vi "SUB-FILE-Measurement data_Save.vi"(0 "File Server Path":string="C:\\InLCT\\Measurement Data\\WB1", 1 "File Name":string="C:\\InLCT\\Measurement Data\\WB1", 2 "배열-열헤더":string[](array[string])=["1", "1", "1", "1", "1", "1", "1", "1"], 3 "배열-Data":dbl[][](array[numeric])=[[30.4, 28.4, 28.4, 28.4, 28.4, 28.4, 28.4, 28.4, 28.4, 28.4, 28.4, 28.4, 28.4, 28.4, 28.4, 28.4, 28.4, 28.4, 28.4, 28.4, 28.4, 28.4, 28.4, 28.4, 28.4, 28.4, 28.4, 28.4, 28.4, 28.4, 28.4, 28.4, 28.4, 28.4, 28.4, 28.4, 28.4, 28.4, 28.4, 28.4, 28.4, 28.4, 28.4, 28.4, 28.4, 28.4, 28.4, 28.4, 28.4, 28.4, 28.4, 28.4, 28.4, 28.4, 28.4, 28.4, 28.4, 28.4, 28.4, 28.4, 28.4, 28.4, 28.4, 28.4, 28.4, 28.4, 28.4, 28.4, 28.4, 28.4, 28.4, 28.4, 28.4, 28.4, 28.4, 28.4, 28.4, 28.4, 28.4, 28.4, 28.4, 28.4, 28.4, 28.4, 28.4, 28.4, 28.4, 28.4, 28.4, 28.4, 28.4, 28.4, 28.4, 28.4, 28.4, 28.4, 28.4, 28.4, 28.4, 28.4, 28.4, 28.4, 28.4, 28.4, 28.4, 28.4, 28.4, 28.4, 28.4, 28.4, 28.4, 28.4, 28.4, 28.4, 28.4, 28.4, 28.4, 28.4, 28.4, 28.4, 28.4, 28.4, 28.4, 28.4, 28.4, 28.4, 28.4, 28.4, 28.4, 28.4, 28.4, 28.4, 28.4, 28.4, 28.4, 28.4, 28.4, 28.4, 28.4, 28.4, 28.4, 28.4, 28.4, 28.4, 28.4, 28.4, 28.4, 28.4, 28.4, 28.4, 28.4, 28.4, 28.4, 28.4, 28.4, 28.4, 28.4, 28.4, 28.4, 28.4, 28.4, 28.4, 28.4, 28.4, 28.4, 28.4, 28.4, 28.4, 28.4, 28.4, 28.4, 28.4, 28.4, 28.4, 28.4, 28.4, 28.4, 28.4, 28.4, 28.4, 28.4, 28.4, 28.4, 28.4, 28.4, 28.4, 28.4, 28.4, 28.4, 28.4, 28.4, 28.4, 28.4, 28.4, 28.4, 28.4, 28.4, 28.4, 28.4, 28.4, 28.4, 28.4, 28.4, 28.4, 28.4, 28.4, 28.4, 28.4, 28.4, 28.4, 28.4, 28.4, 28.4, 28.4, 28.4, 28.4, 28.4, 28.4, 28.4, 28.4, 28.4, 28.4, 28.4, 28.4, 28.4, 28.4, 28.4, 28.4, 28.4, 28.4, 28.4, 28.4, 28.4, 28.4, 28.4, 28.4, 28.4, 28.4, 28.4, 28.4, 28.4, 28.4, 28.4, 28.4, 28.4, 28.4, 28.4, 28.4, 28.4, 28.4, 28.4, 28.4, 28.4, 28.4, 28.4, 28.4, 28.4, 28.4, 28.4, 28.4, 28.4, 28.4, 28.4, 28.4, 28.4, 28.4, 28.4, 28.4, 28.4, 28.4, 28.4, 28.4, 28.4, 28.4, 28.4, 28.4, 28.4, 28.4, 28.4, 28.4, 28.4, 28.4, 28.4, 28.4, 28.4, 28.4, 28.4, 28.4], [28.4, 28.4, 28.4, 28.4, 28.4, 28.4, 28.4, 28.4, 28.4, 28.4, 28.4, 28.4, 28.4, 28.4, 28.4, 28.4, 28.4, 28.4, 28.4, 28.4, 28.4, 28.4, 28.4, 28.4, 28.4, 28.4, 28.4, 28.4, 28.4, 28.4, 28.4, 28.4, 28.4, 28.4, 28.4, 28.4, 28.4, 28.4, 28.4, 28.4, 28.4, 28.4, 28.4, 28.4, 28.4, 28.4, 28.4, 28.4, 28.4, 28.4, 28.4, 28.4, 28.4, 28.4, 28.4, 28.4, 28.4, 28.4, 28.4, 28.4, 28.4, 28.4, 28.4, 28.4, 28.4, 28.4, 28.4, 28.4, 28.4, 28.4, 28.4, 28.4, 28.4, 28.4, 28.4, 28.4, 28.4, 28.4, 28.4, 28.4, 28.4, 28.4, 28.4, 28.4, 28.4, 28.4, 28.4, 28.4, 28.4, 28.4, 28.4, 28.4, 28.4, 28.4, 28.4, 28.4, 28.4, 28.4, 28.4, 28.4, 28.4, 28.4, 28.4, 28.4, 28.4, 28.4, 28.4, 28.4, 28.4, 28.4, 28.4, 28.4, 28.4, 28.4, 28.4, 28.4, 28.4, 28.4, 28.4, 28.4, 28.4, 28.4, 28.4, 28.4, 28.4, 28.4, 28.4, 28.4, 28.4, 28.4, 28.4, 28.4, 28.4, 28.4, 28.4, 28.4, 28.4, 28.4, 28.4, 28.4, 28.4, 28.4, 28.4, 28.4, 28.4, 28.4, 28.4, 28.4, 28.4, 28.4, 28.4, 28.4, 28.4, 28.4, 28.4, 28.4, 28.4, 28.4, 28.4, 28.4, 28.4, 28.4, 28.4, 28.4, 28.4, 28.4, 28.4, 28.4, 28.4, 28.4, 28.4, 28.4, 28.4, 28.4, 28.4, 28.4, 28.4, 28.4, 28.4, 28.4, 28.4, 28.4, 28.4, 28.4, 28.4, 28.4, 28.4, 28.4, 28.4, 28.4, 28.4, 28.4, 28.4, 28.4, 28.4, 28.4, 28.4, 28.4, 28.4, 28.4, 28.4, 28.4, 28.4, 28.4, 28.4, 28.4, 28.4, 28.4, 28.4, 28.4, 28.4, 28.4, 28.4, 28.4, 28.4, 28.4, 28.4, 28.4, 28.4, 28.4, 28.4, 28.4, 28.4, 28.4, 28.4, 28.4, 28.4, 28.4, 28.4, 28.4, 28.4, 28.4, 28.4, 28.4, 28.4, 28.4, 28.4, 28.4, 28.4, 28.4, 28.4, 28.4, 28.4, 28.4, 28.4, 28.4, 28.4, 28.4, 28.4, 28.4, 28.4, 28.4, 28.4, 28.4, 28.4, 28.4, 28.4, 28.4, 28.4, 28.4, 28.4, 28.4, 28.4, 28.4, 28.4, 28.4, 28.4, 28.4, 28.4, 28.4, 28.4, 28.4, 28.4, 28.4, 28.4, 28.4, 28.4, 28.4, 28.4, 28.4, 28.4, 28.4, 28.4, 28.4, 28.4, 28.4, 28.4, 28.4], [28.4, 28.4, 28.4, 28.4, 28.4, 28.4, 28.4, 28.4, 28.4, 28.4, 28.4, 28.4, 28.4, 28.4, 28.4, 28.4, 28.4, 28.4, 28.4, 28.4, 28.4, 28.4, 28.4, 28.4, 28.4, 28.4, 28.4, 28.4, 28.4, 28.4, 28.4, 28.4, 28.4, 28.4, 28.4, 28.4, 28.4, 28.4, 28.4, 28.4, 28.4, 28.4, 28.4, 28.4, 28.4, 28.4, 28.4, 28.4, 28.4, 28.4, 28.4, 28.4, 28.4, 28.4, 28.4, 28.4, 28.4, 28.4, 28.4, 28.4, 28.4, 28.4, 28.4, 28.4, 28.4, 28.4, 28.4, 28.4, 28.4, 28.4, 28.4, 28.4, 28.4, 28.4, 28.4, 28.4, 28.4, 28.4, 28.4, 28.4, 28.4, 28.4, 28.4, 28.4, 28.4, 28.4, 28.4, 28.4, 28.4, 28.4, 28.4, 28.4, 28.4, 28.4, 28.4, 28.4, 28.4, 28.4, 28.4, 28.4, 28.4, 28.4, 28.4, 28.4, 28.4, 28.4, 28.4, 28.4, 28.4, 28.4, 28.4, 28.4, 28.4, 28.4, 28.4, 28.4, 28.4, 28.4, 28.4, 28.4, 28.4, 28.4, 28.4, 28.4, 28.4, 28.4, 28.4, 28.4, 28.4, 28.4, 28.4, 28.4, 28.4, 28.4, 28.4, 28.4, 28.4, 28.4, 28.4, 28.4, 28.4, 28.4, 28.4, 28.4, 28.4, 28.4, 28.4, 28.4, 28.4, 28.4, 28.4, 28.4, 28.4, 28.4, 28.4, 28.4, 28.4, 28.4, 28.4, 28.4, 28.4, 28.4, 28.4, 28.4, 28.4, 28.4, 28.4, 28.4, 28.4, 28.4, 28.4, 28.4, 28.4, 28.4, 28.4, 28.4, 28.4, 28.4, 28.4, 28.4, 28.4, 28.4, 28.4, 28.4, 28.4, 28.4, 28.4, 28.4, 28.4, 28.4, 28.4, 28.4, 28.4, 28.4, 28.4, 28.4, 28.4, 28.4, 28.4, 28.4, 28.4, 28.4, 28.4, 28.4, 28.4, 28.4, 28.4, 28.4, 28.4, 28.4, 28.4, 28.4, 28.4, 28.4, 28.4, 28.4, 28.4, 28.4, 28.4, 28.4, 28.4, 28.4, 28.4, 28.4, 28.4, 28.4, 28.4, 28.4, 28.4, 28.4, 28.4, 28.4, 28.4, 28.4, 28.4, 28.4, 28.4, 28.4, 28.4, 28.4, 28.4, 28.4, 28.4, 28.4, 28.4, 28.4, 28.4, 28.4, 28.4, 28.4, 28.4, 28.4, 28.4, 28.4, 28.4, 28.4, 28.4, 28.4, 28.4, 28.4, 28.4, 28.4, 28.4, 28.4, 28.4, 28.4, 28.4, 28.4, 28.4, 28.4, 28.4, 28.4, 28.4, 28.4, 28.4, 28.4, 28.4, 28.4, 28.4, 28.4, 28.4, 28.4, 28.4, 28.4, 28.4, 28.4, 28.4, 28.4], [28.4, 28.4, 28.4, 28.4, 28.4, 28.4, 28.4, 28.4, 28.4, 28.4, 28.4, 28.4, 28.4, 28.4, 28.4, 28.4, 28.4, 28.4, 28.4, 28.4, 28.4, 28.4, 28.4, 28.4, 28.4, 28.4, 28.4, 28.4, 28.4, 28.4, 28.4, 28.4, 28.4, 28.4, 28.4, 28.4, 28.4, 28.4, 28.4, 28.4, 28.4, 28.4, 28.4, 28.4, 28.4, 28.4, 28.4, 28.4, 28.4, 28.4, 28.4, 28.4, 28.4, 28.4, 28.4, 28.4, 28.4, 28.4, 28.4, 28.4, 28.4, 28.4, 28.4, 28.4, 28.4, 28.4, 28.4, 28.4, 28.4, 28.4, 28.4, 28.4, 28.4, 28.4, 28.4, 28.4, 28.4, 28.4, 28.4, 28.4, 28.4, 28.4, 28.4, 28.4, 28.4, 28.4, 28.4, 28.4, 28.4, 28.4, 28.4, 28.4, 28.4, 28.4, 28.4, 28.4, 28.4, 28.4, 28.4, 28.4, 28.4, 28.4, 28.4, 28.4, 28.4, 28.4, 28.4, 28.4, 28.4, 28.4, 28.4, 28.4, 28.4, 28.4, 28.4, 28.4, 28.4, 28.4, 28.4, 28.4, 28.4, 28.4, 28.4, 28.4, 28.4, 28.4, 28.4, 28.4, 28.4, 28.4, 28.4, 28.4, 28.4, 28.4, 28.4, 28.4, 28.4, 28.4, 28.4, 28.4, 28.4, 28.4, 28.4, 28.4, 28.4, 28.4, 28.4, 28.4, 28.4, 28.4, 28.4, 28.4, 28.4, 28.4, 28.4, 28.4, 28.4, 28.4, 28.4, 28.4, 28.4, 28.4, 28.4, 28.4, 28.4, 28.4, 28.4, 28.4, 28.4, 28.4, 28.4, 28.4, 28.4, 28.4, 28.4, 28.4, 28.4, 28.4, 28.4, 28.4, 28.4, 28.4, 28.4, 28.4, 28.4, 28.4, 28.4, 28.4, 28.4, 28.4, 28.4, 28.4, 28.4, 28.4, 28.4, 28.4, 28.4, 28.4, 28.4, 28.4, 28.4, 28.4, 28.4, 28.4, 28.4, 28.4, 28.4, 28.4, 28.4, 28.4, 28.4, 28.4, 28.4, 28.4, 28.4, 28.4, 28.4, 28.4, 28.4, 28.4, 28.4, 28.4, 28.4, 28.4, 28.4, 28.4, 28.4, 28.4, 28.4, 28.4, 28.4, 28.4, 28.4, 28.4, 28.4, 28.4, 28.4, 28.4, 28.4, 28.4, 28.4, 28.4, 28.4, 28.4, 28.4, 28.4, 28.4, 28.4, 28.4, 28.4, 28.4, 28.4, 28.4, 28.4, 28.4, 28.4, 28.4, 28.4, 28.4, 28.4, 28.4, 28.4, 28.4, 28.4, 28.4, 28.4, 28.4, 28.4, 28.4, 28.4, 28.4, 28.4, 28.4, 28.4, 28.4, 28.4, 28.4, 28.4, 28.4, 28.4, 28.4, 28.4, 28.4, 28.4, 28.4, 28.4, 28.4, 28.4], [28.4, 28.4, 28.4, 28.4, 28.4, 28.4, 28.4, 28.4, 28.4, 28.4, 28.4, 28.4, 28.4, 28.4, 28.4, 28.4, 28.4, 28.4, 28.4, 28.4, 28.4, 28.4, 28.4, 28.4, 28.4, 28.4, 28.4, 28.4, 28.4, 28.4, 28.4, 28.4, 28.4, 28.4, 28.4, 28.4, 28.4, 28.4, 28.4, 28.4, 28.4, 28.4, 28.4, 28.4, 28.4, 28.4, 28.4, 28.4, 28.4, 28.4, 28.4, 28.4, 28.4, 28.4, 28.4, 28.4, 28.4, 28.4, 28.4, 28.4, 28.4, 28.4, 28.4, 28.4, 28.4, 28.4, 28.4, 28.4, 28.4, 28.4, 28.4, 28.4, 28.4, 28.4, 28.4, 28.4, 28.4, 28.4, 28.4, 28.4, 28.4, 28.4, 28.4, 28.4, 28.4, 28.4, 28.4, 28.4, 28.4, 28.4, 28.4, 28.4, 28.4, 28.4, 28.4, 28.4, 28.4, 28.4, 28.4, 28.4, 28.4, 28.4, 28.4, 28.4, 28.4, 28.4, 28.4, 28.4, 28.4, 28.4, 28.4, 28.4, 28.4, 28.4, 28.4, 28.4, 28.4, 28.4, 28.4, 28.4, 28.4, 28.4, 28.4, 28.4, 28.4, 28.4, 28.4, 28.4, 28.4, 28.4, 28.4, 28.4, 28.4, 28.4, 28.4, 28.4, 28.4, 28.4, 28.4, 28.4, 28.4, 28.4, 28.4, 28.4, 28.4, 28.4, 28.4, 28.4, 28.4, 28.4, 28.4, 28.4, 28.4, 28.4, 28.4, 28.4, 28.4, 28.4, 28.4, 28.4, 28.4, 28.4, 28.4, 28.4, 28.4, 28.4, 28.4, 28.4, 28.4, 28.4, 28.4, 28.4, 28.4, 28.4, 28.4, 28.4, 28.4, 28.4, 28.4, 28.4, 28.4, 28.4, 28.4, 28.4, 28.4, 28.4, 28.4, 28.4, 28.4, 28.4, 28.4, 28.4, 28.4, 28.4, 28.4, 28.4, 28.4, 28.4, 28.4, 28.4, 28.4, 28.4, 28.4, 28.4, 28.4, 28.4, 28.4, 28.4, 28.4, 28.4, 28.4, 28.4, 28.4, 28.4, 28.4, 28.4, 28.4, 28.4, 28.4, 28.4, 28.4, 28.4, 28.4, 28.4, 28.4, 28.4, 28.4, 28.4, 28.4, 28.4, 28.4, 28.4, 28.4, 28.4, 28.4, 28.4, 28.4, 28.4, 28.4, 28.4, 28.4, 28.4, 28.4, 28.4, 28.4, 28.4, 28.4, 28.4, 28.4, 28.4, 28.4, 28.4, 28.4, 28.4, 28.4, 28.4, 28.4, 28.4, 28.4, 28.4, 28.4, 28.4, 28.4, 28.4, 28.4, 28.4, 28.4, 28.4, 28.4, 28.4, 28.4, 28.4, 28.4, 28.4, 28.4, 28.4, 28.4, 28.4, 28.4, 28.4, 28.4, 28.4, 28.4, 28.4, 28.4, 28.4, 28.4, 28.4], [28.4, 28.4, 28.4, 28.4, 28.4, 28.4, 28.4, 28.4, 28.4, 28.4, 28.4, 28.4, 28.4, 28.4, 28.4, 28.4, 28.4, 28.4, 28.4, 28.4, 28.4, 28.4, 28.4, 28.4, 28.4, 28.4, 28.4, 28.4, 28.4, 28.4, 28.4, 28.4, 28.4, 28.4, 28.4, 28.4, 28.4, 28.4, 28.4, 28.4, 28.4, 28.4, 28.4, 28.4, 28.4, 28.4, 28.4, 28.4, 28.4, 28.4, 28.4, 28.4, 28.4, 28.4, 28.4, 28.4, 28.4, 28.4, 28.4, 28.4, 28.4, 28.4, 28.4, 28.4, 28.4, 28.4, 28.4, 28.4, 28.4, 28.4, 28.4, 28.4, 28.4, 28.4, 28.4, 28.4, 28.4, 28.4, 28.4, 28.4, 28.4, 28.4, 28.4, 28.4, 28.4, 28.4, 28.4, 28.4, 28.4, 28.4, 28.4, 28.4, 28.4, 28.4, 28.4, 28.4, 28.4, 28.4, 28.4, 28.4, 28.4, 28.4, 28.4, 28.4, 28.4, 28.4, 28.4, 28.4, 28.4, 28.4, 28.4, 28.4, 28.4, 28.4, 28.4, 28.4, 28.4, 28.4, 28.4, 28.4, 28.4, 28.4, 28.4, 28.4, 28.4, 28.4, 28.4, 28.4, 28.4, 28.4, 28.4, 28.4, 28.4, 28.4, 28.4, 28.4, 28.4, 28.4, 28.4, 28.4, 28.4, 28.4, 28.4, 28.4, 28.4, 28.4, 28.4, 28.4, 28.4, 28.4, 28.4, 28.4, 28.4, 28.4, 28.4, 28.4, 28.4, 28.4, 28.4, 28.4, 28.4, 28.4, 28.4, 28.4, 28.4, 28.4, 28.4, 28.4, 28.4, 28.4, 28.4, 28.4, 28.4, 28.4, 28.4, 28.4, 28.4, 28.4, 28.4, 28.4, 28.4, 28.4, 28.4, 28.4, 28.4, 28.4, 28.4, 28.4, 28.4, 28.4, 28.4, 28.4, 28.4, 28.4, 28.4, 28.4, 28.4, 28.4, 28.4, 28.4, 28.4, 28.4, 28.4, 28.4, 28.4, 28.4, 28.4, 28.4, 28.4, 28.4, 28.4, 28.4, 28.4, 28.4, 28.4, 28.4, 28.4, 28.4, 28.4, 28.4, 28.4, 28.4, 28.4, 28.4, 28.4, 28.4, 28.4, 28.4, 28.4, 28.4, 28.4, 28.4, 28.4, 28.4, 28.4, 28.4, 28.4, 28.4, 28.4, 28.4, 28.4, 28.4, 28.4, 28.4, 28.4, 28.4, 28.4, 28.4, 28.4, 28.4, 28.4, 28.4, 28.4, 28.4, 28.4, 28.4, 28.4, 28.4, 28.4, 28.4, 28.4, 28.4, 28.4, 28.4, 28.4, 28.4, 28.4, 28.4, 28.4, 28.4, 28.4, 28.4, 28.4, 28.4, 28.4, 28.4, 28.4, 28.4, 28.4, 28.4, 28.4, 28.4, 28.4, 28.4, 28.4, 28.4, 28.4, 28.4], [28.4, 28.4, 28.4, 28.4, 28.4, 28.4, 28.4, 28.4, 28.4, 28.4, 28.4, 28.4, 28.4, 28.4, 28.4, 28.4, 28.4, 28.4, 28.4, 28.4, 28.4, 28.4, 28.4, 28.4, 28.4, 28.4, 28.4, 28.4, 28.4, 28.4, 28.4, 28.4, 28.4, 28.4, 28.4, 28.4, 28.4, 28.4, 28.4, 28.4, 28.4, 28.4, 28.4, 28.4, 28.4, 28.4, 28.4, 28.4, 28.4, 28.4, 28.4, 28.4, 28.4, 28.4, 28.4, 28.4, 28.4, 28.4, 28.4, 28.4, 28.4, 28.4, 28.4, 28.4, 28.4, 28.4, 28.4, 28.4, 28.4, 28.4, 28.4, 28.4, 28.4, 28.4, 28.4, 28.4, 28.4, 28.4, 28.4, 28.4, 28.4, 28.4, 28.4, 28.4, 28.4, 28.4, 28.4, 28.4, 28.4, 28.4, 28.4, 28.4, 28.4, 28.4, 28.4, 28.4, 28.4, 28.4, 28.4, 28.4, 28.4, 28.4, 28.4, 28.4, 28.4, 28.4, 28.4, 28.4, 28.4, 28.4, 28.4, 28.4, 28.4, 28.4, 28.4, 28.4, 28.4, 28.4, 28.4, 28.4, 28.4, 28.4, 28.4, 28.4, 28.4, 28.4, 28.4, 28.4, 28.4, 28.4, 28.4, 28.4, 28.4, 28.4, 28.4, 28.4, 28.4, 28.4, 28.4, 28.4, 28.4, 28.4, 28.4, 28.4, 28.4, 28.4, 28.4, 28.4, 28.4, 28.4, 28.4, 28.4, 28.4, 28.4, 28.4, 28.4, 28.4, 28.4, 28.4, 28.4, 28.4, 28.4, 28.4, 28.4, 28.4, 28.4, 28.4, 28.4, 28.4, 28.4, 28.4, 28.4, 28.4, 28.4, 28.4, 28.4, 28.4, 28.4, 28.4, 28.4, 28.4, 28.4, 28.4, 28.4, 28.4, 28.4, 28.4, 28.4, 28.4, 28.4, 28.4, 28.4, 28.4, 28.4, 28.4, 28.4, 28.4, 28.4, 28.4, 28.4, 28.4, 28.4, 28.4, 28.4, 28.4, 28.4, 28.4, 28.4, 28.4, 28.4, 28.4, 28.4, 28.4, 28.4, 28.4, 28.4, 28.4, 28.4, 28.4, 28.4, 28.4, 28.4, 28.4, 28.4, 28.4, 28.4, 28.4, 28.4, 28.4, 28.4, 28.4, 28.4, 28.4, 28.4, 28.4, 28.4, 28.4, 28.4, 28.4, 28.4, 28.4, 28.4, 28.4, 28.4, 28.4, 28.4, 28.4, 28.4, 28.4, 28.4, 28.4, 28.4, 28.4, 28.4, 28.4, 28.4, 28.4, 28.4, 28.4, 28.4, 28.4, 28.4, 28.4, 28.4, 28.4, 28.4, 28.4, 28.4, 28.4, 28.4, 28.4, 28.4, 28.4, 28.4, 28.4, 28.4, 28.4, 28.4, 28.4, 28.4, 28.4, 28.4, 28.4, 28.4, 28.4, 28.4, 28.4, 28.4], [28.4, 28.4, 28.4, 28.4, 28.4, 28.4, 28.4, 28.4, 28.4, 28.4, 28.4, 28.4, 28.4, 28.4, 28.4, 28.4, 28.4, 28.4, 28.4, 28.4, 28.4, 28.4, 28.4, 28.4, 28.4, 28.4, 28.4, 28.4, 28.4, 28.4, 28.4, 28.4, 28.4, 28.4, 28.4, 28.4, 28.4, 28.4, 28.4, 28.4, 28.4, 28.4, 28.4, 28.4, 28.4, 28.4, 28.4, 28.4, 28.4, 28.4, 28.4, 28.4, 28.4, 28.4, 28.4, 28.4, 28.4, 28.4, 28.4, 28.4, 28.4, 28.4, 28.4, 28.4, 28.4, 28.4, 28.4, 28.4, 28.4, 28.4, 28.4, 28.4, 28.4, 28.4, 28.4, 28.4, 28.4, 28.4, 28.4, 28.4, 28.4, 28.4, 28.4, 28.4, 28.4, 28.4, 28.4, 28.4, 28.4, 28.4, 28.4, 28.4, 28.4, 28.4, 28.4, 28.4, 28.4, 28.4, 28.4, 28.4, 28.4, 28.4, 28.4, 28.4, 28.4, 28.4, 28.4, 28.4, 28.4, 28.4, 28.4, 28.4, 28.4, 28.4, 28.4, 28.4, 28.4, 28.4, 28.4, 28.4, 28.4, 28.4, 28.4, 28.4, 28.4, 28.4, 28.4, 28.4, 28.4, 28.4, 28.4, 28.4, 28.4, 28.4, 28.4, 28.4, 28.4, 28.4, 28.4, 28.4, 28.4, 28.4, 28.4, 28.4, 28.4, 28.4, 28.4, 28.4, 28.4, 28.4, 28.4, 28.4, 28.4, 28.4, 28.4, 28.4, 28.4, 28.4, 28.4, 28.4, 28.4, 28.4, 28.4, 28.4, 28.4, 28.4, 28.4, 28.4, 28.4, 28.4, 28.4, 28.4, 28.4, 28.4, 28.4, 28.4, 28.4, 28.4, 28.4, 28.4, 28.4, 28.4, 28.4, 28.4, 28.4, 28.4, 28.4, 28.4, 28.4, 28.4, 28.4, 28.4, 28.4, 28.4, 28.4, 28.4, 28.4, 28.4, 28.4, 28.4, 28.4, 28.4, 28.4, 28.4, 28.4, 28.4, 28.4, 28.4, 28.4, 28.4, 28.4, 28.4, 28.4, 28.4, 28.4, 28.4, 28.4, 28.4, 28.4, 28.4, 28.4, 28.4, 28.4, 28.4, 28.4, 28.4, 28.4, 28.4, 28.4, 28.4, 28.4, 28.4, 28.4, 28.4, 28.4, 28.4, 28.4, 28.4, 28.4, 28.4, 28.4, 28.4, 28.4, 28.4, 28.4, 28.4, 28.4, 28.4, 28.4, 28.4, 28.4, 28.4, 28.4, 28.4, 28.4, 28.4, 28.4, 28.4, 28.4, 28.4, 28.4, 28.4, 28.4, 28.4, 28.4, 28.4, 28.4, 28.4, 28.4, 28.4, 28.4, 28.4, 28.4, 28.4, 28.4, 28.4, 28.4, 28.4, 28.4, 28.4, 28.4, 28.4, 28.4, 28.4, 28.4, 28.4, 28.4, 28.4]], 4 "precision (6)":i16) -> (5 "정상(T)":bool caption="정상", 6 "Path":string)   [LabVIEW 2015]
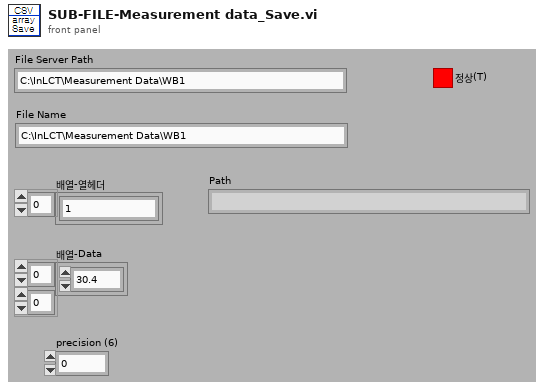
[diagram p1: front panel]
types:
  T1 = enum16{"open", "replace", "create", "open or create", "replace or create", "replace or create with confirmation"}
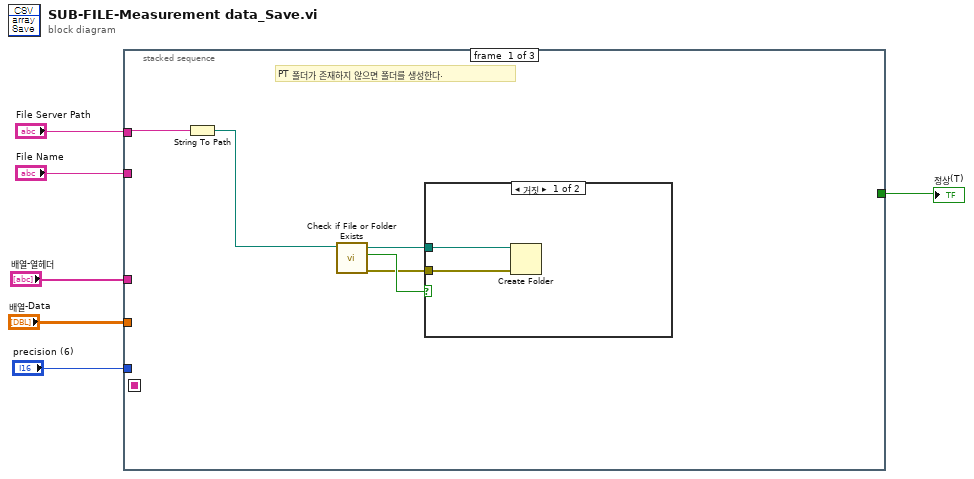
[diagram p0: block diagram]
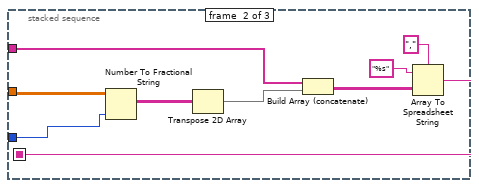
[diagram p3: hidden frame]
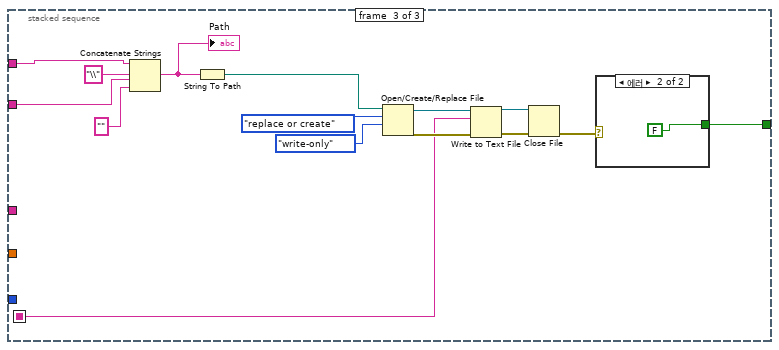
[diagram p4: hidden frame]
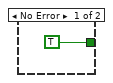
[diagram p5: hidden frame]
diagram:
  n1 = stacked-sequence {
    seq-local: [_ w17 _] -> [_ _ w24]
    tunnel: "배열-Data" -> [_ w22 _]
    tunnel: "배열-열헤더" -> [_ w21 _]
    tunnel: "File Server Path" -> [w11 _ w29]
    tunnel: "File Name" -> [_ _ w28]
    tunnel: [_ _ w25] -> w2
    tunnel: "precision (6)" -> [_ w14 _]
    frame #0 {
      # "PT 폴더가 존재하지 않으면 폴더를 생성한다."
      n2 = String To Path(string=w11) -> (path=w10:path)
      n3 = call <vilib>:"Check if File or Folder Exists.vi"("path"=w10) -> ("error out"=w8:errorcluster, "file or folder exists?"=w9:bool, "dup path"=w7:path)  [unwired: 8 in]
      n4 = case shown="거짓" w9 {
        tunnel: w8 -> [w13 _]
        tunnel: w7 -> [w12 _]
        frame False {
          n5 = Create Folder(path (use dialog)=w12, error in=w13) -> ()  [unwired: 1 in, 3 out]
        }
        frame True {
        }
      }
    }
    frame #1 {
      n6 = Number To Fractional String(number=w22, precision (6)=w14) -> (F-format string=w16:string[][])  [unwired: 2 in]
      n7 = Transpose 2D Array(2D array=w16) -> (transposed array=w15:string[][])
      n8 = Build Array (concatenate)(w21, w15) -> (w20:string[][])
      n9 = Array To Spreadsheet String(delimiter (Tab)="," ("구분 문자(탭)"), array=w20, 3:"%s" ("포맷 문자열")) -> (spreadsheet string=w17:string)
    }
    frame #2 {
      n10 = Concatenate Strings(w29, "\\" ("format (%.3f)"), w28, "" ("format (%.3f)")) -> (w30:string)
      "Path" <- w30
      n11 = String To Path(string=w30) -> (path=w27:path)
      n12 = Open/Create/Replace File(file path (use dialog)=w27, operation (0:open)=T1."replace or create" ("동작(0:open)"), access (0:read/write)=enum16{"read/write", "read-only", "write-only"}."write-only" ("접근(0:읽기/쓰기)")) -> (refnum out=w33:refnum<file>, error out=w32:errorcluster)  [unwired: 1 in, 3 out]
      n13 = Write to Text File(file (use dialog)=w33, text=w24, error in=w32) -> (refnum out=w34:refnum<file>, error out=w35:errorcluster)  [unwired: 2 out]
      n14 = Close File(refnum=w34, error in=w35) -> (error out=w26:errorcluster)  [unwired: 1 out]
      n15 = case shown="에러" w26 {
        tunnel: [TRUE FALSE] -> w25
        frame No Error {
        }
        frame Error {
        }
      }
    }
  }
  "정상(T)" <- w2
